vi "Facade.vi"(0 "Data In":T4, 2 "Display State In":T2={"华氏?"=FALSE, "显示模式开关？"=TRUE}, 3 "Container State":T3) -> (6 "Data Out":T4, 7 "Display State Out":T2={"华氏?"=FALSE, "显示模式开关？"=TRUE}, 8 "Action":T1)   [LabVIEW 2011, in "双模温度计2.xctl"]
uses:
  Data.ctl
  <vilib>/_xctls/Container State.ctl
  State.ctl
  <vilib>/_xctls/Action.ctl
  <vilib>/_xctls/XControlSupport.lvlib
panel:
  in  "Boolean":bool
  out "Thermometer":dbl(slide) scale=0.0..100.0
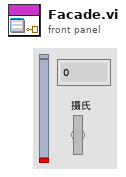
[diagram p1: front panel]
types:
  T1 = typedef "XControlSupport.lvlib/Action.ctl" = cluster{"Data Changed?":bool, "State Changed?":bool, "Action Name":string}
  T2 = typedef "双模温度计2.xctl/State.ctl" = cluster{"华氏?":bool, "显示模式开关？":bool}
  T3 = typedef "XControlSupport.lvlib/Container State.ctl" = cluster{"Indicator?":bool, "Run Mode?":bool, " Refnum":refnum<vi>}
  T4 = typedef "双模温度计2.xctl/Data.ctl" = dbl
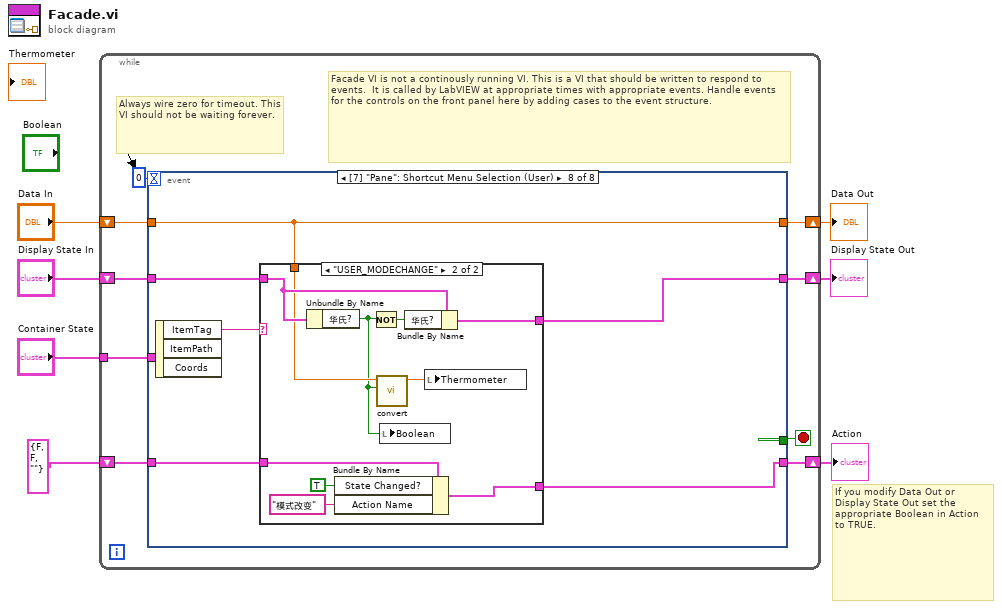
[diagram p0: block diagram]
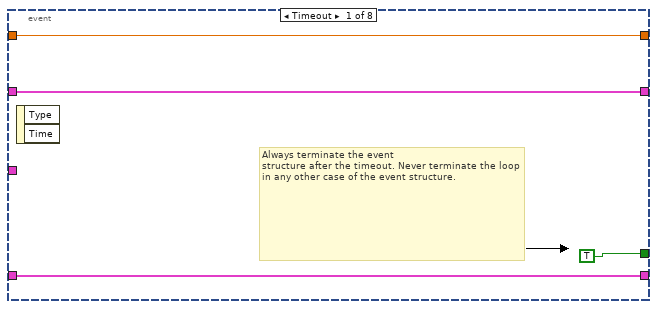
[diagram p2: hidden frame]
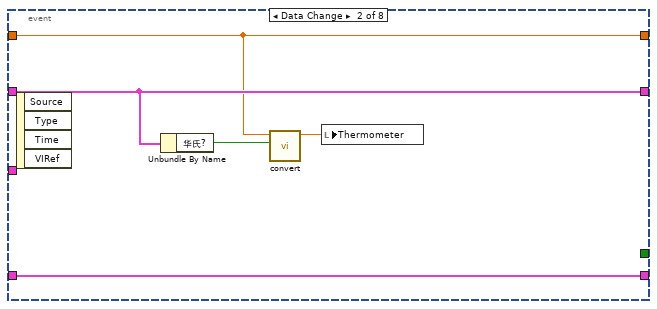
[diagram p3: hidden frame]
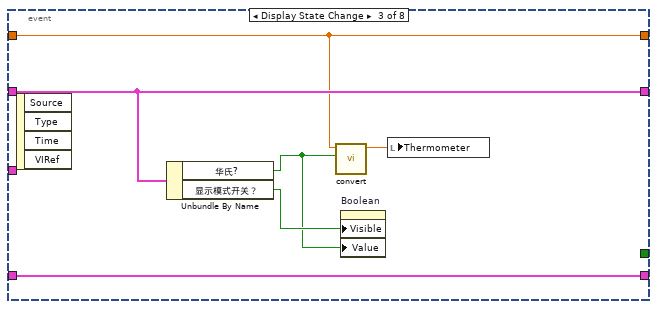
[diagram p4: hidden frame]
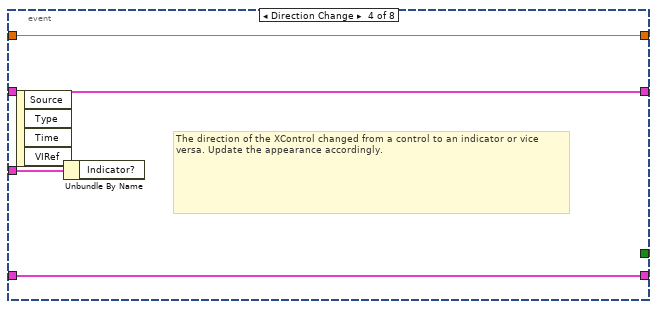
[diagram p5: hidden frame]
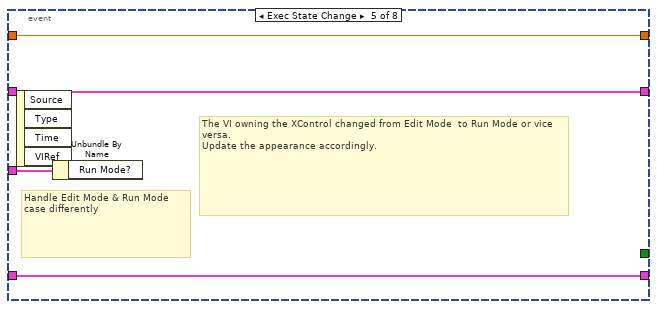
[diagram p6: hidden frame]
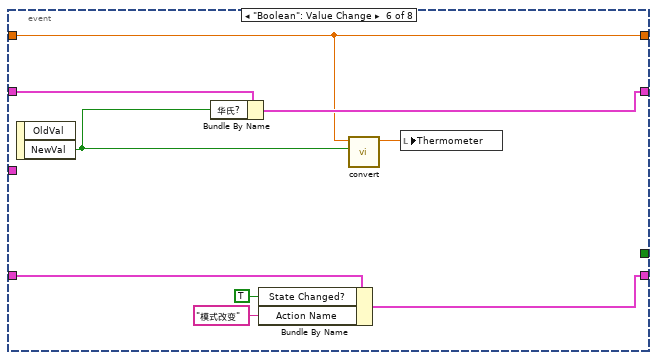
[diagram p7: hidden frame]
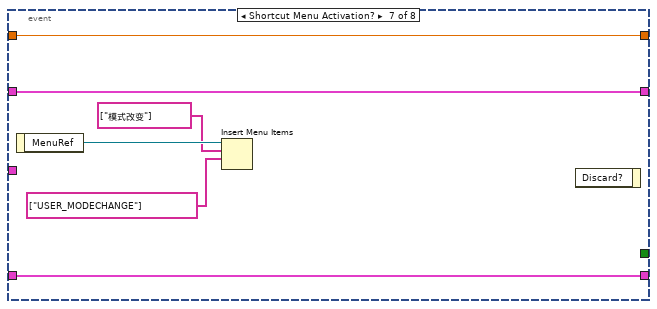
[diagram p8: hidden frame]
diagram:
  # "If you modify Data Out or\nDisplay State Out set the\nappropriate Boolean in Action\nto TRUE."
  n1 = while {
    shift-right: [w15] -> w4
    shift-left: "Display State In" -> [w16]
    tunnel: "Container State" -> [w12]
    shift-right: [w10] -> w7
    shift-left: "Data In" -> [w11]
    shift-right: [w8] -> w2
    shift-left: T1 {"Data Changed?"=FALSE, "State Changed?"=FALSE, "Action Name"=""} ("Action") -> [w9]
    stop <- w14 stop-if-true
    # "Facade VI is not a continously running VI. This is a VI that should be written to respond to events.  It is called by LabVIEW at appropriate times with appropriate events. Handle events for the controls on the front panel here by adding cases to the event structure."
    # "Always wire zero for timeout. This\nVI should not be waiting forever."
    n2 = event shown="[7] \"Pane\": Shortcut Menu Selection (User)" {
      selector: _ -> [_ _ _ _ _ _ _ _]
      dyn-events: _ -> [_ _ _ _ _ _ _ _]
      timeout: 0 -> [_ _ _ _ _ _ _ _]
      tunnel: w16 -> [w18 w24 w30 w34 w38 w48 w53 w59]
      tunnel: [w18 w24 w30 w34 w38 w47 w53 w58] -> w15
      tunnel: [TRUE _ _ _ _ _ _ _] -> w14
      tunnel: w12 -> [_ _ _ w35 w39 _ _ _]
      tunnel: w11 -> [w17 w22 w28 w33 w37 w45 w54 w56]
      tunnel: [w17 w22 w28 w33 w37 w45 w54 w56] -> w10
      tunnel: [w19 w25 w31 w32 w36 w42 w52 w55] -> w8
      tunnel: w9 -> [w19 w25 w31 w32 w36 w43 w52 w57]
      event Timeout {
        # "Always terminate the event\nstructure after the timeout. Never terminate the loop in any other case of the event structure."
        n3 = event-data() -> ()  [unwired: 1 in, 2 out]
      }
      event Data Change {
        n4 = event-data() -> ()  [unwired: 1 in, 4 out]
        n5 = Unbundle By Name(w24) -> ("华氏?"=w23:bool)
        n6 = call "convert.vi"("华氏?"=w23, "Data In in"=w22) -> ("Data In out"=w21:T4)  [unwired: 9 in]
        n7 = local write "Thermometer"(w21) -> ()
      }
      event Display State Change {
        n8 = event-data() -> ()  [unwired: 1 in, 4 out]
        n9 = Unbundle By Name(w30) -> ("华氏?"=w26:bool, "显示模式开关？"=w27:bool)
        n10 = call "convert.vi"("华氏?"=w26, "Data In in"=w28) -> ("Data In out"=w29:T4)  [unwired: 9 in]
        n11 = property on="Boolean" class="Bool (strict)"("Visible"=w27, "Value"=w26) -> ()  [unwired: 2 in, 2 out]
        n12 = local write "Thermometer"(w29) -> ()
      }
      event Direction Change {
        # "The direction of the XControl changed from a control to an indicator or vice versa. Update the appearance accordingly."
        n13 = event-data() -> ()  [unwired: 1 in, 4 out]
        n14 = Unbundle By Name(w35) -> ()  [unwired: 1 out]
      }
      event Exec State Change {
        # "The VI owning the XControl changed from Edit Mode  to Run Mode or vice versa.\nUpdate the appearance accordingly."
        # "Handle Edit Mode & Run Mode\ncase differently"
        n15 = event-data() -> ()  [unwired: 1 in, 4 out]
        n16 = Unbundle By Name(w39) -> ()  [unwired: 1 out]
      }
      event "Boolean": Value Change {
        n17 = event-data() -> ("NewVal"=w44:bool)  [unwired: 1 in, 1 out]
        n18 = Bundle By Name(cluster=w48, "华氏?"=w44) -> (w47:T2)
        n19 = Bundle By Name(cluster=w43, "State Changed?"=TRUE, "Action Name"="模式改变") -> (w42:T1)
        n20 = call "convert.vi"("华氏?"=w44, "Data In in"=w45) -> ("Data In out"=w46:T4)  [unwired: 9 in]
        n21 = local write "Thermometer"(w46) -> ()
      }
      event Shortcut Menu Activation? {
        n22 = event-data() -> ("MenuRef"=w51:refnum<k9>)  [unwired: 1 in]
        n23 = Insert Menu Items(7:string[] ["USER_MODECHANGE"] ("item tags"), 8:string[] ["模式改变"] ("item names"), 9:w51) -> ()  [unwired: 3 in, 3 out]
        n24 = event-data() -> ()  [unwired: 2 in, 1 out]
      }
      event Shortcut Menu Selection (User) {
        n25 = event-data() -> ("ItemTag"=w60:string)  [unwired: 1 in, 2 out]
        n26 = case shown="\"USER_MODECHANGE\"" w60 {
          tunnel: w59 -> [w62 w72]
          tunnel: [w62 w70] -> w58
          tunnel: w57 -> [w61 w67]
          tunnel: w56 -> [_ w68]
          tunnel: [w61 w66] -> w55
          frame "False", Default {
          }
          frame "USER_MODECHANGE" {
            n27 = Unbundle By Name(w72) -> ("华氏?"=w63:bool)
            n28 = Bundle By Name(cluster=w67, "State Changed?"=TRUE, "Action Name"="模式改变") -> (w66:T1)
            n29 = Not(x=w63) -> (.not. x?=w71:bool)
            n30 = call "convert.vi"("华氏?"=w63, "Data In in"=w68) -> ("Data In out"=w69:T4)  [unwired: 9 in]
            n31 = local write "Boolean"(w63) -> ()
            n32 = Bundle By Name(cluster=w72, "华氏?"=w71) -> (w70:T2)
            n33 = local write "Thermometer"(w69) -> ()
          }
        }
      }
    }
  }
  "Display State Out" <- w4
  "Data Out" <- w7
  "Action" <- w2
